vi "VISJS Viewer.vi"(4 "Extra Scripts":string, 5 "FileDependency out":map{path, T1}(c390), 6 "Options":string, 7 "OpenWebBrowser(False)":bool, 8 "error in":errorcluster, 9 "Embedd VISJS Librarya in HTMl File(False)":bool, 10 "HTMLFilePath":path, 11 "LibraryDependency":map{path, T3}(c390)) -> (0 "error out":errorcluster, 3 "HTMLFileContent":string)   [LabVIEW 2020, in "VISJS Viewer.lvlib"] (continued)
=e||\"Set\"===e)return Uo(g);if(\"Arguments\"===e||/^(?:Ui|I)nt(?:8|16|32)(?:Clamped)?Array$/.test(e))return rP(g,t)}(g))||t&&g&&\"number\"==typeof g.length){A&&(g=A);var e=0,C=function(){};return{s:C,n:function(){return e>=g.length?{done:!0}:{done:!1,value:g[e++]}},e:function(g){throw g},f:C}}throw new TypeError(\"Invalid attempt to iterate non-iterable instance.\\nIn order to be iterable, non-array objects must have a [Symbol.iterator]() method.\")}var I,i=!0,o=!1;return{s:function(){A=A.call(g)},n:function(){var g=A.next();return i=g.done,g},e:function(g){o=!0,I=g},f:function(){try{i||null==A.return||A.return()}finally{if(o)throw I}}}}function rP(g,t){(null==t||t>g.length)&&(t=g.length);for(var A=0,e=new Array(t);A<t;A++)e[A]=g[A];return e}var sP=function(){function g(t,A,e){var C,I,i,o,n,r,s,a,d,h,l,c,u;cn(this,g),this.body=t,this.canvas=A,this.selectionHandler=e,this.navigationHandler=new oP(t,A),this.body.eventListeners.onTap=je(C=this.onTap).call(C,this),this.body.eventListeners.onTouch=je(I=this.onTouch).call(I,this),this.body.eventListeners.onDoubleTap=je(i=this.onDoubleTap).call(i,this),this.body.eventListeners.onHold=je(o=this.onHold).call(o,this),this.body.eventListeners.onDragStart=je(n=this.onDragStart).call(n,this),this.body.eventListeners.onDrag=je(r=this.onDrag).call(r,this),this.body.eventListeners.onDragEnd=je(s=this.onDragEnd).call(s,this),this.body.eventListeners.onMouseWheel=je(a=this.onMouseWheel).call(a,this),this.body.eventListeners.onPinch=je(d=this.onPinch).call(d,this),this.body.eventListeners.onMouseMove=je(h=this.onMouseMove).call(h,this),this.body.eventListeners.onRelease=je(l=this.onRelease).call(l,this),this.body.eventListeners.onContext=je(c=this.onContext).call(c,this),this.touchTime=0,this.drag={},this.pinch={},this.popup=void 0,this.popupObj=void 0,this.popupTimer=void 0,this.body.functions.getPointer=je(u=this.getPointer).call(u,this),this.options={},this.defaultOptions={dragNodes:!0,dragView:!0,hover:!1,keyboard:{enabled:!1,speed:{x:10,y:10,zoom:.02},bindToWindow:!0,autoFocus:!0},navigationButtons:!1,tooltipDelay:300,zoomView:!0,zoomSpeed:1},fe(this.options,this.defaultOptions),this.bindEventListeners()}return kd(g,[{key:\"bindEventListeners\",value:function(){var g=this;this.body.emitter.on(\"destroy\",(function(){clearTimeout(g.popupTimer),delete g.body.functions.getPointer}))}},{key:\"setOptions\",value:function(g){if(void 0!==g){Jf([\"hideEdgesOnDrag\",\"hideEdgesOnZoom\",\"hideNodesOnDrag\",\"keyboard\",\"multiselect\",\"selectable\",\"selectConnectedEdges\"],this.options,g),dv(this.options,g,\"keyboard\"),g.tooltip&&(fe(this.options.tooltip,g.tooltip),g.tooltip.color&&(this.options.tooltip.color=Iv(g.tooltip.color)))}this.navigationHandler.setOptions(this.options)}},{key:\"getPointer\",value:function(g){return{x:g.x-(t=this.canvas.frame.canvas,t.getBoundingClientRect().left),y:g.y-gv(this.canvas.frame.canvas)};var t}},{key:\"onTouch\",value:function(g){(new Date).valueOf()-this.touchTime>50&&(this.drag.pointer=this.getPointer(g.center),this.drag.pinched=!1,this.pinch.scale=this.body.view.scale,this.touchTime=(new Date).valueOf())}},{key:\"onTap\",value:function(g){var t=this.getPointer(g.center),A=this.selectionHandler.options.multiselect&&(g.changedPointers[0].ctrlKey||g.changedPointers[0].metaKey);this.checkSelectionChanges(t,A),this.selectionHandler.commitAndEmit(t,g),this.selectionHandler.generateClickEvent(\"click\",g,t)}},{key:\"onDoubleTap\",value:function(g){var t=this.getPointer(g.center);this.selectionHandler.generateClickEvent(\"doubleClick\",g,t)}},{key:\"onHold\",value:function(g){var t=this.getPointer(g.center),A=this.selectionHandler.options.multiselect;this.checkSelectionChanges(t,A),this.selectionHandler.commitAndEmit(t,g),this.selectionHandler.generateClickEvent(\"click\",g,t),this.selectionHandler.generateClickEvent(\"hold\",g,t)}},{key:\"onRelease\",value:function(g){if((new Date).valueOf()-this.touchTime>10){var t=this.getPointer(g.center);this.selectionHandler.generateClickEvent(\"release\",g,t),this.touchTime=(new Date).valueOf()}}},{key:\"onContext\",value:function(g){var t=this.getPointer({x:g.clientX,y:g.clientY});this.selectionHandler.generateClickEvent(\"oncontext\",g,t)}},{key:\"checkSelectionChanges\",value:function(g){!0===(arguments.length>1&&void 0!==arguments[1]&&arguments[1])?this.selectionHandler.selectAdditionalOnPoint(g):this.selectionHandler.selectOnPoint(g)}},{key:\"_determineDifference\",value:function(g,t){var A=function(g,t){for(var A=[],e=0;e<g.length;e++){var C=g[e];-1===Xc(t).call(t,C)&&A.push(C)}return A};return{nodes:A(g.nodes,t.nodes),edges:A(g.edges,t.edges)}}},{key:\"onDragStart\",value:function(g){if(!this.drag.dragging){void 0===this.drag.pointer&&this.onTouch(g);var t=this.selectionHandler.getNodeAt(this.drag.pointer);if(this.drag.dragging=!0,this.drag.selection=[],this.drag.translation=fe({},this.body.view.translation),this.drag.nodeId=void 0,g.srcEvent.shiftKey){this.body.selectionBox.show=!0;var A=this.getPointer(g.center);this.body.selectionBox.position.start={x:this.canvas._XconvertDOMtoCanvas(A.x),y:this.canvas._YconvertDOMtoCanvas(A.y)},this.body.selectionBox.position.end={x:this.canvas._XconvertDOMtoCanvas(A.x),y:this.canvas._YconvertDOMtoCanvas(A.y)}}else if(void 0!==t&&!0===this.options.dragNodes){this.drag.nodeId=t.id,!1===t.isSelected()&&this.selectionHandler.setSelection({nodes:[t.id]}),this.selectionHandler.generateClickEvent(\"dragStart\",g,this.drag.pointer);var e,C=nP(this.selectionHandler.getSelectedNodes());try{for(C.s();!(e=C.n()).done;){var I=e.value,i={id:I.id,node:I,x:I.x,y:I.y,xFixed:I.options.fixed.x,yFixed:I.options.fixed.y};I.options.fixed.x=!0,I.options.fixed.y=!0,this.drag.selection.push(i)}}catch(g){C.e(g)}finally{C.f()}}else this.selectionHandler.generateClickEvent(\"dragStart\",g,this.drag.pointer,void 0,!0)}}},{key:\"onDrag\",value:function(g){var t=this;if(!0!==this.drag.pinched){this.body.emitter.emit(\"unlockNode\");var A=this.getPointer(g.center),e=this.drag.selection;if(e&&e.length&&!0===this.options.dragNodes){this.selectionHandler.generateClickEvent(\"dragging\",g,A);var C=A.x-this.drag.pointer.x,I=A.y-this.drag.pointer.y;Cl(e).call(e,(function(g){var A=g.node;!1===g.xFixed&&(A.x=t.canvas._XconvertDOMtoCanvas(t.canvas._XconvertCanvasToDOM(g.x)+C)),!1===g.yFixed&&(A.y=t.canvas._YconvertDOMtoCanvas(t.canvas._YconvertCanvasToDOM(g.y)+I))})),this.body.emitter.emit(\"startSimulation\")}else{if(g.srcEvent.shiftKey){if(this.selectionHandler.generateClickEvent(\"dragging\",g,A,void 0,!0),void 0===this.drag.pointer)return void this.onDragStart(g);this.body.selectionBox.position.end={x:this.canvas._XconvertDOMtoCanvas(A.x),y:this.canvas._YconvertDOMtoCanvas(A.y)},this.body.emitter.emit(\"_requestRedraw\")}if(!0===this.options.dragView&&!g.srcEvent.shiftKey){if(this.selectionHandler.generateClickEvent(\"dragging\",g,A,void 0,!0),void 0===this.drag.pointer)return void this.onDragStart(g);var i=A.x-this.drag.pointer.x,o=A.y-this.drag.pointer.y;this.body.view.translation={x:this.drag.translation.x+i,y:this.drag.translation.y+o},this.body.emitter.emit(\"_requestRedraw\")}}}}},{key:\"onDragEnd\",value:function(g){var t=this;if(this.drag.dragging=!1,this.body.selectionBox.show){var A;this.body.selectionBox.show=!1;var e=this.body.selectionBox.position,C={minX:Math.min(e.start.x,e.end.x),minY:Math.min(e.start.y,e.end.y),maxX:Math.max(e.start.x,e.end.x),maxY:Math.max(e.start.y,e.end.y)},I=pc(A=this.body.nodeIndices).call(A,(function(g){var A=t.body.nodes[g];return A.x>=C.minX&&A.x<=C.maxX&&A.y>=C.minY&&A.y<=C.maxY}));Cl(I).call(I,(function(g){return t.selectionHandler.selectObject(t.body.nodes[g])}));var i=this.getPointer(g.center);this.selectionHandler.commitAndEmit(i,g),this.selectionHandler.generateClickEvent(\"dragEnd\",g,this.getPointer(g.center),void 0,!0),this.body.emitter.emit(\"_requestRedraw\")}else{var o=this.drag.selection;o&&o.length?(Cl(o).call(o,(function(g){g.node.options.fixed.x=g.xFixed,g.node.options.fixed.y=g.yFixed})),this.selectionHandler.generateClickEvent(\"dragEnd\",g,this.getPointer(g.center)),this.body.emitter.emit(\"startSimulation\")):(this.selectionHandler.generateClickEvent(\"dragEnd\",g,this.getPointer(g.center),void 0,!0),this.body.emitter.emit(\"_requestRedraw\"))}}},{key:\"onPinch\",value:function(g){var t=this.getPointer(g.center);this.drag.pinched=!0,void 0===this.pinch.scale&&(this.pinch.scale=1);var A=this.pinch.scale*g.scale;this.zoom(A,t)}},{key:\"zoom\",value:function(g,t){if(!0===this.options.zoomView){var A=this.body.view.scale;g<1e-5&&(g=1e-5),g>10&&(g=10);var e=void 0;void 0!==this.drag&&!0===this.drag.dragging&&(e=this.canvas.DOMtoCanvas(this.drag.pointer));var C=this.body.view.translation,I=g/A,i=(1-I)*t.x+C.x*I,o=(1-I)*t.y+C.y*I;if(this.body.view.scale=g,this.body.view.translation={x:i,y:o},null!=e){var n=this.canvas.canvasToDOM(e);this.drag.pointer.x=n.x,this.drag.pointer.y=n.y}this.body.emitter.emit(\"_requestRedraw\"),A<g?this.body.emitter.emit(\"zoom\",{direction:\"+\",scale:this.body.view.scale,pointer:t}):this.body.emitter.emit(\"zoom\",{direction:\"-\",scale:this.body.view.scale,pointer:t})}}},{key:\"onMouseWheel\",value:function(g){if(!0===this.options.zoomView){if(0!==g.deltaY){var t=this.body.view.scale;t*=1+(g.deltaY<0?1:-1)*(.1*this.options.zoomSpeed);var A=this.getPointer({x:g.clientX,y:g.clientY});this.zoom(t,A)}g.preventDefault()}}},{key:\"onMouseMove\",value:function(g){var t=this,A=this.getPointer({x:g.clientX,y:g.clientY}),e=!1;void 0!==this.popup&&(!1===this.popup.hidden&&this._checkHidePopup(A),!1===this.popup.hidden&&(e=!0,this.popup.setPosition(A.x+3,A.y-5),this.popup.show())),this.options.keyboard.autoFocus&&!1===this.options.keyboard.bindToWindow&&!0===this.options.keyboard.enabled&&this.canvas.frame.focus(),!1===e&&(void 0!==this.popupTimer&&(clearInterval(this.popupTimer),this.popupTimer=void 0),this.drag.dragging||(this.popupTimer=wu((function(){return t._checkShowPopup(A)}),this.options.tooltipDelay))),!0===this.options.hover&&this.selectionHandler.hoverObject(g,A)}},{key:\"_checkShowPopup\",value:function(g){var t=this.canvas._XconvertDOMtoCanvas(g.x),A=this.canvas._YconvertDOMtoCanvas(g.y),e={left:t,top:A,right:t,bottom:A},C=void 0===this.popupObj?void 0:this.popupObj.id,I=!1,i=\"node\";if(void 0===this.popupObj){for(var o,n=this.body.nodeIndices,r=this.body.nodes,s=[],a=0;a<n.length;a++)!0===(o=r[n[a]]).isOverlappingWith(e)&&(I=!0,void 0!==o.getTitle()&&s.push(n[a]));s.length>0&&(this.popupObj=r[s[s.length-1]],I=!0)}if(void 0===this.popupObj&&!1===I){for(var d,h=this.body.edgeIndices,l=this.body.edges,c=[],u=0;u<h.length;u++)!0===(d=l[h[u]]).isOverlappingWith(e)&&!0===d.connected&&void 0!==d.getTitle()&&c.push(h[u]);c.length>0&&(this.popupObj=l[c[c.length-1]],i=\"edge\")}void 0!==this.popupObj?this.popupObj.id!==C&&(void 0===this.popup&&(this.popup=new Ov(this.canvas.frame)),this.popup.popupTargetType=i,this.popup.popupTargetId=this.popupObj.id,this.popup.setPosition(g.x+3,g.y-5),this.popup.setText(this.popupObj.getTitle()),this.popup.show(),this.body.emitter.emit(\"showPopup\",this.popupObj.id)):void 0!==this.popup&&(this.popup.hide(),this.body.emitter.emit(\"hidePopup\"))}},{key:\"_checkHidePopup\",value:function(g){var t=this.selectionHandler._pointerToPositionObject(g),A=!1;if(\"node\"===this.popup.popupTargetType){if(void 0!==this.body.nodes[this.popup.popupTargetId]&&!0===(A=this.body.nodes[this.popup.popupTargetId].isOverlappingWith(t))){var e=this.selectionHandler.getNodeAt(g);A=void 0!==e&&e.id===this.popup.popupTargetId}}else void 0===this.selectionHandler.getNodeAt(g)&&void 0!==this.body.edges[this.popup.popupTargetId]&&(A=this.body.edges[this.popup.popupTargetId].isOverlappingWith(t));!1===A&&(this.popupObj=void 0,this.popup.hide(),this.body.emitter.emit(\"hidePopup\"))}}]),g}(),aP=u,dP=pm,hP=zy.getWeakData,lP=qy,cP=AA,uP=Q,pP=gg,fP=Hy,vP=qg,yP=GC.set,mP=GC.getterFor,bP=Sr.find,wP=Sr.findIndex,kP=aP([].splice),xP=0,EP=function(g){return g.frozen||(g.frozen=new OP)},OP=function(){this.entries=[]},TP=function(g,t){return bP(g.entries,(function(g){return g[0]===t}))};OP.prototype={get:function(g){var t=TP(this,g);if(t)return t[1]},has:function(g){return!!TP(this,g)},set:function(g,t){var A=TP(this,g);A?A[1]=t:this.entries.push([g,t])},delete:function(g){var t=wP(this.entries,(function(t){return t[0]===g}));return~t&&kP(this.entries,t,1),!!~t}};var DP,NP={getConstructor:function(g,t,A,e){var C=g((function(g,C){lP(g,I),yP(g,{type:t,id:xP++,frozen:void 0}),uP(C)||fP(C,g[e],{that:g,AS_ENTRIES:A})})),I=C.prototype,i=mP(t),o=function(g,t,A){var e=i(g),C=hP(cP(t),!0);return!0===C?EP(e).set(t,A):C[e.id]=A,g};return dP(I,{delete:function(g){var t=i(this);if(!pP(g))return!1;var A=hP(g);return!0===A?EP(t).delete(g):A&&vP(A,t.id)&&delete A[t.id]},has:function(g){var t=i(this);if(!pP(g))return!1;var A=hP(g);return!0===A?EP(t).has(g):A&&vP(A,t.id)}}),dP(I,A?{get:function(g){var t=i(this);if(pP(g)){var A=hP(g);return!0===A?EP(t).get(g):A?A[t.id]:void 0}},set:function(g,t){return o(this,g,t)}}:{add:function(g){return o(this,g,!0)}}),C}},RP=vy,PP=C,MP=u,BP=pm,zP=zy,SP=cm,ZP=NP,FP=gg,GP=GC.enforce,jP=I,LP=bC,VP=Object,YP=Array.isArray,WP=VP.isExtensible,QP=VP.isFrozen,UP=VP.isSealed,_P=VP.freeze,KP=VP.seal,HP={},XP={},JP=!PP.ActiveXObject&&\"ActiveXObject\"in PP,qP=function(g){return function(){return g(this,arguments.length?arguments[0]:void 0)}},$P=SP(\"WeakMap\",qP,ZP),gM=$P.prototype,tM=MP(gM.set);if(LP)if(JP){DP=ZP.getConstructor(qP,\"WeakMap\",!0),zP.enable();var AM=MP(gM.delete),eM=MP(gM.has),CM=MP(gM.get);BP(gM,{delete:function(g){if(FP(g)&&!WP(g)){var t=GP(this);return t.frozen||(t.frozen=new DP),AM(this,g)||t.frozen.delete(g)}return AM(this,g)},has:function(g){if(FP(g)&&!WP(g)){var t=GP(this);return t.frozen||(t.frozen=new DP),eM(this,g)||t.frozen.has(g)}return eM(this,g)},get:function(g){if(FP(g)&&!WP(g)){var t=GP(this);return t.frozen||(t.frozen=new DP),eM(this,g)?CM(this,g):t.frozen.get(g)}return CM(this,g)},set:function(g,t){if(FP(g)&&!WP(g)){var A=GP(this);A.frozen||(A.frozen=new DP),eM(this,g)?tM(this,g,t):A.frozen.set(g,t)}else tM(this,g,t);return this}})}else RP&&jP((function(){var g=_P([]);return tM(new $P,g,1),!QP(g)}))&&BP(gM,{set:function(g,t){var A;return YP(g)&&(QP(g)?A=HP:UP(g)&&(A=XP)),tM(this,g,t),A===HP&&_P(g),A===XP&&KP(g),this}});var IM,iM,oM,nM,rM,sM=A(tg.WeakMap);function aM(g,t,A,e){if(\"a\"===A&&!e)throw new TypeError(\"Private accessor was defined without a getter\");if(\"function\"==typeof t?g!==t||!e:!t.has(g))throw new TypeError(\"Cannot read private member from an object whose class did not declare it\");return\"m\"===A?e:\"a\"===A?e.call(g):e?e.value:t.get(g)}function dM(g,t,A,e,C){if(\"m\"===e)throw new TypeError(\"Private method is not writable\");if(\"a\"===e&&!C)throw new TypeError(\"Private accessor was defined without a setter\");if(\"function\"==typeof t?g!==t||!C:!t.has(g))throw new TypeError(\"Cannot write private member to an object whose class did not declare it\");return\"a\"===e?C.call(g,A):C?C.value=A:t.set(g,A),A}function hM(g,t){var A=void 0!==uh&&ln(g)||g[\"@@iterator\"];if(!A){if(Rh(g)||(A=function(g,t){var A;if(!g)return;if(\"string\"==typeof g)return lM(g,t);var e=wh(A=Object.prototype.toString.call(g)).call(A,8,-1);\"Object\"===e&&g.constructor&&(e=g.constructor.name);if(\"Map\"===e||\"Set\"===e)return Uo(g);if(\"Arguments\"===e||/^(?:Ui|I)nt(?:8|16|32)(?:Clamped)?Array$/.test(e))return lM(g,t)}(g))||t&&g&&\"number\"==typeof g.length){A&&(g=A);var e=0,C=function(){};return{s:C,n:function(){return e>=g.length?{done:!0}:{done:!1,value:g[e++]}},e:function(g){throw g},f:C}}throw new TypeError(\"Invalid attempt to iterate non-iterable instance.\\nIn order to be iterable, non-array objects must have a [Symbol.iterator]() method.\")}var I,i=!0,o=!1;return{s:function(){A=A.call(g)},n:function(){var g=A.next();return i=g.done,g},e:function(g){o=!0,I=g},f:function(){try{i||null==A.return||A.return()}finally{if(o)throw I}}}}function lM(g,t){(null==t||t>g.length)&&(t=g.length);for(var A=0,e=new Array(t);A<t;A++)e[A]=g[A];return e}function cM(g,t){var A,e=new CO,C=hM(t);try{for(C.s();!(A=C.n()).done;){var I=A.value;g.has(I)||e.add(I)}}catch(g){C.e(g)}finally{C.f()}return e}\"function\"==typeof SuppressedError&&SuppressedError;var uM=function(){function g(){cn(this,g),IM.set(this,new CO),iM.set(this,new CO)}return kd(g,[{key:\"size\",get:function(){return aM(this,iM,\"f\").size}},{key:\"add\",value:function(){for(var g=arguments.length,t=new Array(g),A=0;A<g;A++)t[A]=arguments[A];for(var e=0,C=t;e<C.length;e++){var I=C[e];aM(this,iM,\"f\").add(I)}}},{key:\"delete\",value:function(){for(var g=arguments.length,t=new Array(g),A=0;A<g;A++)t[A]=arguments[A];for(var e=0,C=t;e<C.length;e++){var I=C[e];aM(this,iM,\"f\").delete(I)}}},{key:\"clear\",value:function(){aM(this,iM,\"f\").clear()}},{key:\"getSelection\",value:function(){return ch(aM(this,iM,\"f\"))}},{key:\"getChanges\",value:function(){return{added:ch(cM(aM(this,IM,\"f\"),aM(this,iM,\"f\"))),deleted:ch(cM(aM(this,iM,\"f\"),aM(this,IM,\"f\"))),previous:ch(new CO(aM(this,IM,\"f\"))),current:ch(new CO(aM(this,iM,\"f\")))}}},{key:\"commit\",value:function(){var g=this.getChanges();dM(this,IM,aM(this,iM,\"f\"),\"f\"),dM(this,iM,new CO(aM(this,IM,\"f\")),\"f\");var t,A=hM(g.added);try{for(A.s();!(t=A.n()).done;){t.value.select()}}catch(g){A.e(g)}finally{A.f()}var e,C=hM(g.deleted);try{for(C.s();!(e=C.n()).done;){e.value.unselect()}}catch(g){C.e(g)}finally{C.f()}return g}}]),g}();IM=new sM,iM=new sM;var pM=function(){function g(){var t=arguments.length>0&&void 0!==arguments[0]?arguments[0]:function(){};cn(this,g),oM.set(this,new uM),nM.set(this,new uM),rM.set(this,void 0),dM(this,rM,t,\"f\")}return kd(g,[{key:\"sizeNodes\",get:function(){return aM(this,oM,\"f\").size}},{key:\"sizeEdges\",get:function(){return aM(this,nM,\"f\").size}},{key:\"getNodes\",value:function(){return aM(this,oM,\"f\").getSelection()}},{key:\"getEdges\",value:function(){return aM(this,nM,\"f\").getSelection()}},{key:\"addNodes\",value:function(){var g;(g=aM(this,oM,\"f\")).add.apply(g,arguments)}},{key:\"addEdges\",value:function(){var g;(g=aM(this,nM,\"f\")).add.apply(g,arguments)}},{key:\"deleteNodes\",value:function(g){aM(this,oM,\"f\").delete(g)}},{key:\"deleteEdges\",value:function(g){aM(this,nM,\"f\").delete(g)}},{key:\"clear\",value:function(){aM(this,oM,\"f\").clear(),aM(this,nM,\"f\").clear()}},{key:\"commit\",value:function(){for(var g,t,A={nodes:aM(this,oM,\"f\").commit(),edges:aM(this,nM,\"f\").commit()},e=arguments.length,C=new Array(e),I=0;I<e;I++)C[I]=arguments[I];return(g=aM(this,rM,\"f\")).call.apply(g,bh(t=[this,A]).call(t,C)),A}}]),g}();function fM(g,t){var A=void 0!==uh&&ln(g)||g[\"@@iterator\"];if(!A){if(Rh(g)||(A=function(g,t){var A;if(!g)return;if(\"string\"==typeof g)return vM(g,t);var e=wh(A=Object.prototype.toString.call(g)).call(A,8,-1);\"Object\"===e&&g.constructor&&(e=g.constructor.name);if(\"Map\"===e||\"Set\"===e)return Uo(g);if(\"Arguments\"===e||/^(?:Ui|I)nt(?:8|16|32)(?:Clamped)?Array$/.test(e))return vM(g,t)}(g))||t&&g&&\"number\"==typeof g.length){A&&(g=A);var e=0,C=function(){};return{s:C,n:function(){return e>=g.length?{done:!0}:{done:!1,value:g[e++]}},e:function(g){throw g},f:C}}throw new TypeError(\"Invalid attempt to iterate non-iterable instance.\\nIn order to be iterable, non-array objects must have a [Symbol.iterator]() method.\")}var I,i=!0,o=!1;return{s:function(){A=A.call(g)},n:function(){var g=A.next();return i=g.done,g},e:function(g){o=!0,I=g},f:function(){try{i||null==A.return||A.return()}finally{if(o)throw I}}}}function vM(g,t){(null==t||t>g.length)&&(t=g.length);for(var A=0,e=new Array(t);A<t;A++)e[A]=g[A];return e}oM=new sM,nM=new sM,rM=new sM;var yM=function(){function g(t,A){var e=this;cn(this,g),this.body=t,this.canvas=A,this._selectionAccumulator=new pM,this.hoverObj={nodes:{},edges:{}},this.options={},this.defaultOptions={multiselect:!1,selectable:!0,selectConnectedEdges:!0,hoverConnectedEdges:!0},fe(this.options,
